vi "Save Actor DB.vi"(8 "error in (no error)":errorcluster, 10 "Actor DB":variant, 11 "Actor Store":refnum<class "Actor Store.lvclass">) -> (0 "error out":errorcluster, 2 "Actor DB Out":variant, 3 "Actor Store":refnum<class "Actor Store.lvclass">)   [LabVIEW 2023, in "Add Async Methods Actor.lvlib"]
uses:
  Add Async Methods Actor.lvlib
  Classes/Actor Store/Actor Store.lvclass
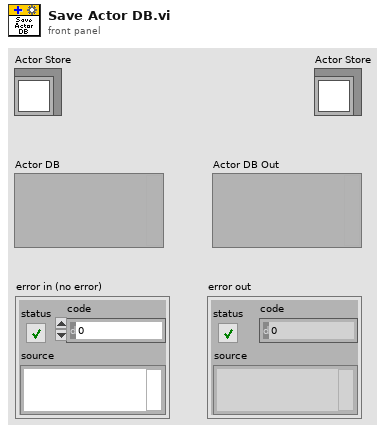
[diagram p1: front panel]
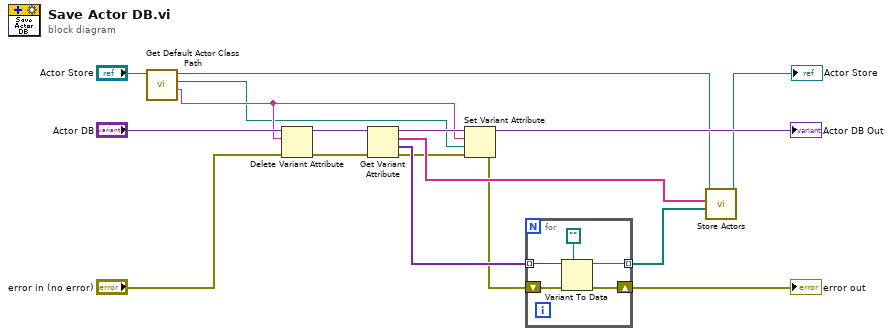
[diagram p0: block diagram]
diagram:
  n1 = call "Get Default Actor Class Path.vi"("Actor Store"="Actor Store") -> ("Actor Label"=w3:string, "Path String"=w2:path, "Actor Store"=w4:refnum<class "Actor Store.lvclass">)  [unwired: 7 in, 1 out]
  n2 = Delete Variant Attribute(4:"error in (no error)", 6:w3, 7:"Actor DB") -> (0:w14:errorcluster, 3:w16:variant)  [unwired: 1 out]
  n3 = Get Variant Attribute(Variant=w16, error in=w14) -> (duplicate Variant=w13:variant, names=w10:string[], values=w11:variant[], error out=w9:errorcluster)  [unwired: 2 in]
  n4 = Set Variant Attribute(Variant=w13, name=w3, value=w2, error in=w9) -> (Variant out=→"Actor DB Out":variant, error out=w8:errorcluster)  [unwired: 1 out]
  n5 = for {
    tunnel: w11 -> [w22] mode=indexing
    shift-right: [w20] -> w7
    shift-left: w8 -> [w19]
    tunnel: [w18] -> w1 mode=indexing
    n6 = Variant To Data(error in=w19, type=path "" ("Path to Actor"), Variant=w22) -> (data=w18:path, error out=w20:errorcluster)
  }
  "error out" <- w7
  n7 = call-dynamic "Store Actors.vi"("Actor Paths"=w1, "Actors"=w10, "Actor Store in"=w4) -> ("Actor Store out"=→"Actor Store":refnum<class "Actor Store.lvclass">)  [unwired: 7 in, 1 out]
